vi "Delete old Files and Check Free Size.vi"() -> ()   [LabVIEW 2014]
panel:
  out "File List":cluster{"last mod":timestamp, path}[](array[cluster])
  out "size(s)":i32
  out "Delete Clicked?":bool
  in  "Delete":bool
  out "Free":dbl
  out "Exceed":bool
  in  "Limit":dbl
  out "free (bytes)":i64
  out "size (bytes)":i64
  # "Delete oldest File"
  # "Free Size Available Check"
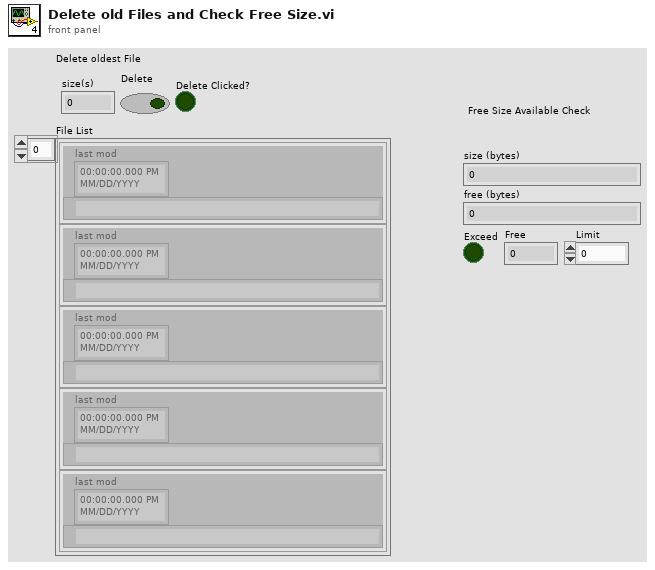
[diagram p1: front panel]
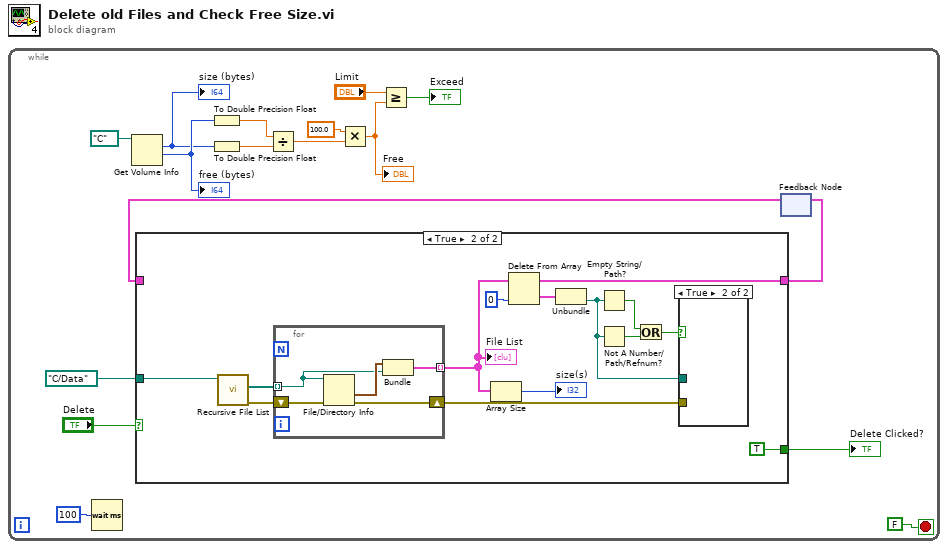
[diagram p0: block diagram]
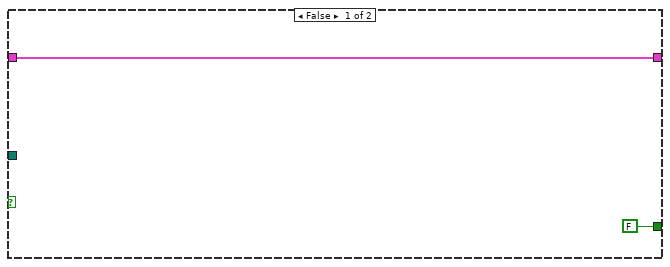
[diagram p2: hidden frame]
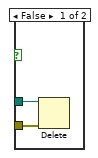
[diagram p3: hidden frame]
diagram:
  n1 = while {
    stop <- FALSE stop-if-true
    n2 = Wait (ms)(milliseconds to wait=u32 100) -> ()  [unwired: 1 out]
    n3 = Get Volume Info(11:path "C:/") -> (1:w16:i64, 2:w15:i64)  [unwired: 1 in, 4 out]
    "size (bytes)" <- w15
    "free (bytes)" <- w16
    n4 = To Double Precision Float(number=w16) -> (double precision float=w12:dbl)
    n5 = To Double Precision Float(number=w15) -> (double precision float=w11:dbl)
    n6 = Divide(x=w12, y=w11) -> (x/y=w14:dbl)
    n7 = Multiply(x=100.0, y=w14) -> (x*y=w8:dbl)
    "Free" <- w8
    n8 = Greater Or Equal?(x="Limit", y=w8) -> (x >= y?=→"Exceed":bool)
    n9 = feedback #1() -> (w1:cluster{"last mod":timestamp, path}[])  [unwired: 1 in]
    n10 = case shown="True" "Delete" {
      tunnel: path "C:/Data" -> [_ w32]
      tunnel: [FALSE TRUE] -> w4
      tunnel: [w18 w27] -> w2
      tunnel: w1 -> [w18 _]
      frame False {
      }
      frame True {
        n11 = call <vilib>:"Recursive File List.vi"("Folder Path"=w32) -> ("error out"=w31:errorcluster, "All Files in Dir"=w33:path[])  [unwired: 6 in, 3 out]
        n12 = for {
          tunnel: w33 -> [w39] mode=indexing
          tunnel: [w38] -> w26 mode=indexing
          shift-right: [w36] -> w24
          shift-left: w31 -> [w37]
          n13 = File/Directory Info(path=w39, error in=w37) -> (last mod=w40:timestamp, error out=w36:errorcluster)  [unwired: 5 out]
          n14 = Bundle("last mod"=w40, w39) -> (w38:cluster{"last mod":timestamp, path})  [unwired: 1 in]
        }
        "File List" <- w26
        n15 = Array Size(array=w26) -> (size(s)=→"size(s)":i32)
        n16 = Delete From Array(array=w26, index=0) -> (deleted portion=w28:cluster{"last mod":timestamp, path}, array with subset deleted=w27:cluster{"last mod":timestamp, path}[])  [unwired: 1 in]
        n17 = Unbundle(w28) -> (w21:path)  [unwired: 1 out]
        n18 = Empty String/Path?(string/path=w21) -> (empty?=w23:bool)
        n19 = Not A Number/Path/Refnum?(number/path/refnum=w21) -> (NaN/Path/Refnum?=w22:bool)
        n20 = Or(x=w23, y=w22) -> (x .or. y?=w20:bool)
        n21 = case shown="True" w20 {
          tunnel: w24 -> [w35 _]
          tunnel: w21 -> [w34 _]
          frame False {
            n22 = Delete(path (use dialog)=w34, error in=w35) -> ()  [unwired: 3 in, 3 out]
          }
          frame True {
          }
        }
      }
    }
    "Delete Clicked?" <- w4
    n23 = feedback-in #1(w2) -> ()
  }
